vi "简易流程调试界面.vi"() -> ()   [LabVIEW 2016, in "斯坦道氨氮.lvlib"]
uses:
  <userlib>/_OpenG.lib/array/array.llb/Sort 1D Array (I32)__ogtk.vi
  <vilib>/Plasmionique/MB Master/MB_Master/MB_Master.lvclass
panel:
  in  "停止":bool
  out "故障状态":string
  out "告警状态":string
  out "工作状态":string
  in  "单步测试":bool
  out "注射器温度":sgl
  out "消解温度":sgl
  out "ADC":sgl
  out "F3":sgl format="%#.6f"
  out "F2":sgl format="%#.6f"
  out "F1":sgl format="%#.6f"
  out "F0":sgl format="%#.6f"
  in  "启动":bool
  in  "简易流程":u16(ring)
  in  "参数下拉列表":u16(ring)
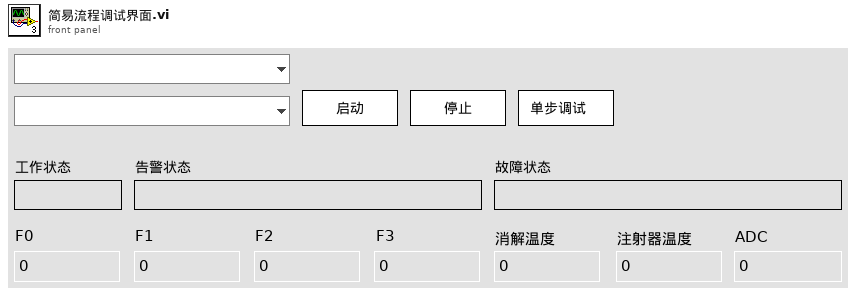
[diagram p1: front panel]
types:
  T1 = typedef "LVStringsAndValuesArrayTypeDef_U16.ctl" = cluster{"String":string, "Value":u16}[]
  T2 = cluster{"系统时间":timestamp, "工作状态":u16, "测量模式":enum16{"待机", "连续模式", "周期模式", "定点模式", "受控模式", "手动模式"}, "告警代码":u16, "故障代码":u16, "日志代码":u16, "软件版本":u16, "F0":sgl, "F1":sgl, "F2":sgl, "F3":sgl, "T":sgl, "H":sgl, "id":u16, "flowid":u16, "量程":u16, "总磷控温温度1":sgl, "营养盐控温温度2":sgl, "ADC":sgl}
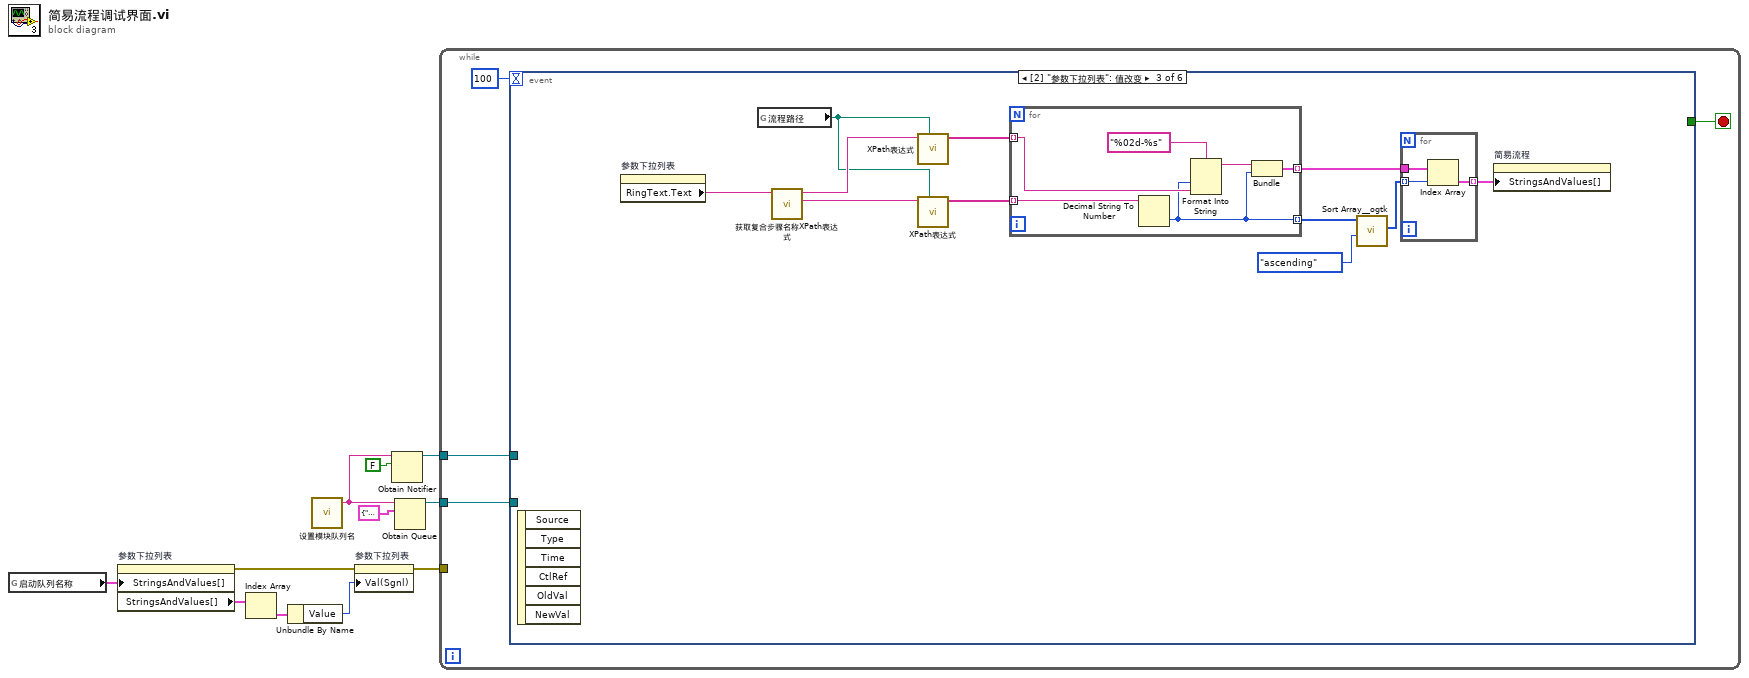
[diagram p0: block diagram]
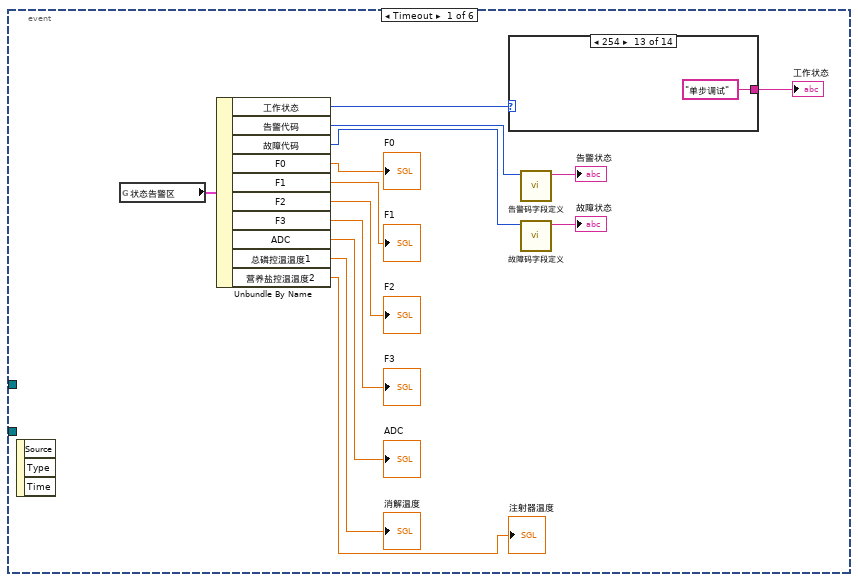
[diagram p2: hidden frame]
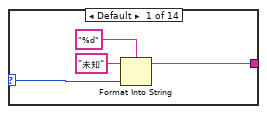
[diagram p3: hidden frame]
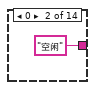
[diagram p4: hidden frame]
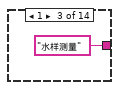
[diagram p5: hidden frame]
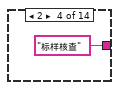
[diagram p6: hidden frame]
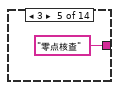
[diagram p7: hidden frame]
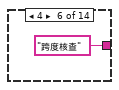
[diagram p8: hidden frame]
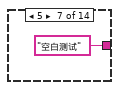
[diagram p9: hidden frame]
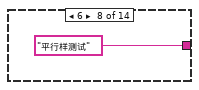
[diagram p10: hidden frame]
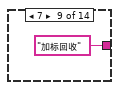
[diagram p11: hidden frame]
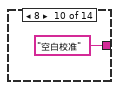
[diagram p12: hidden frame]
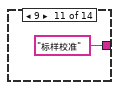
[diagram p13: hidden frame]
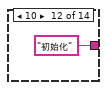
[diagram p14: hidden frame]
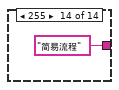
[diagram p15: hidden frame]
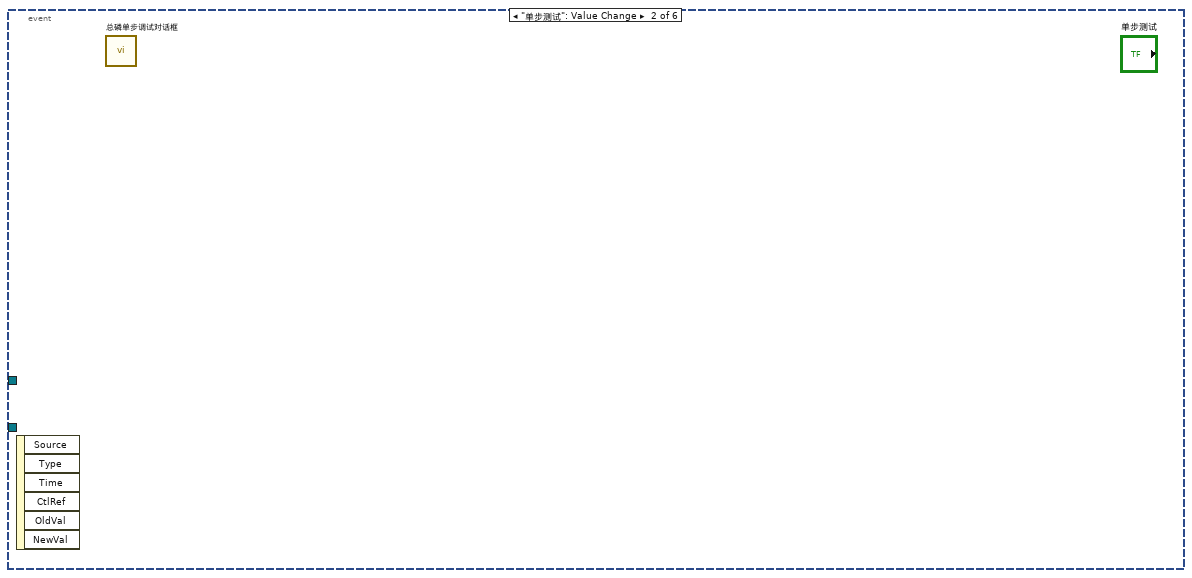
[diagram p16: hidden frame]
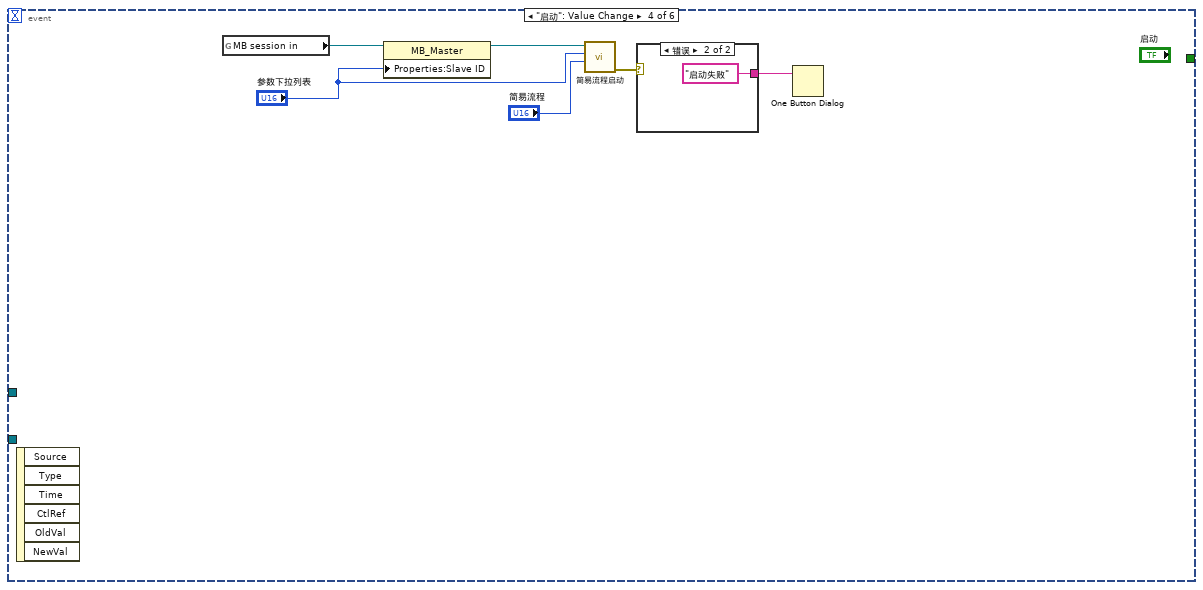
[diagram p17: hidden frame]
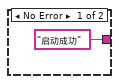
[diagram p18: hidden frame]
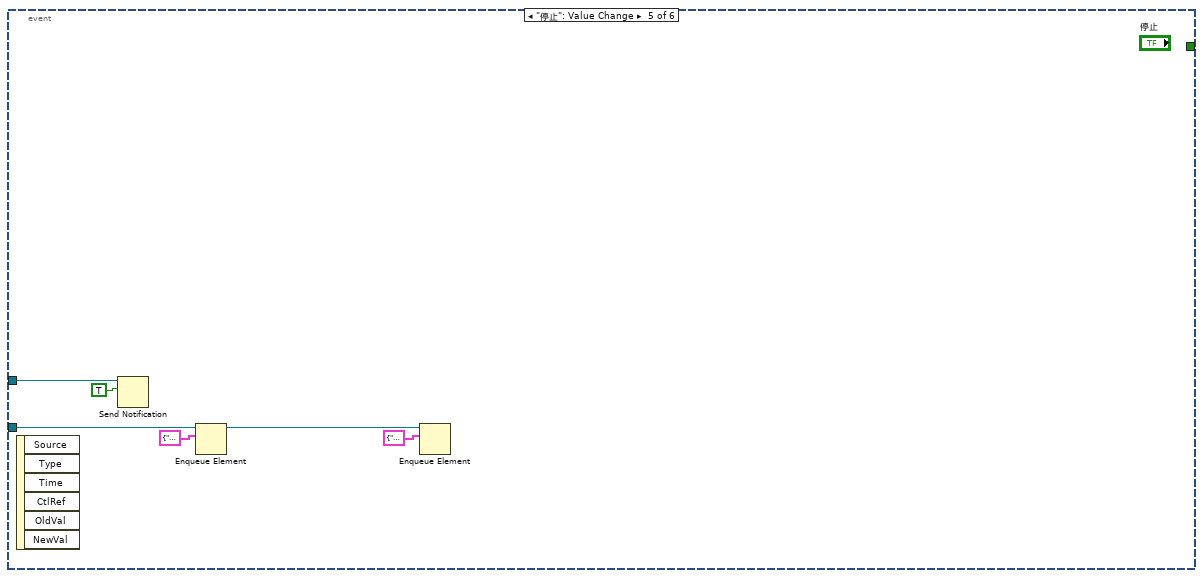
[diagram p19: hidden frame]
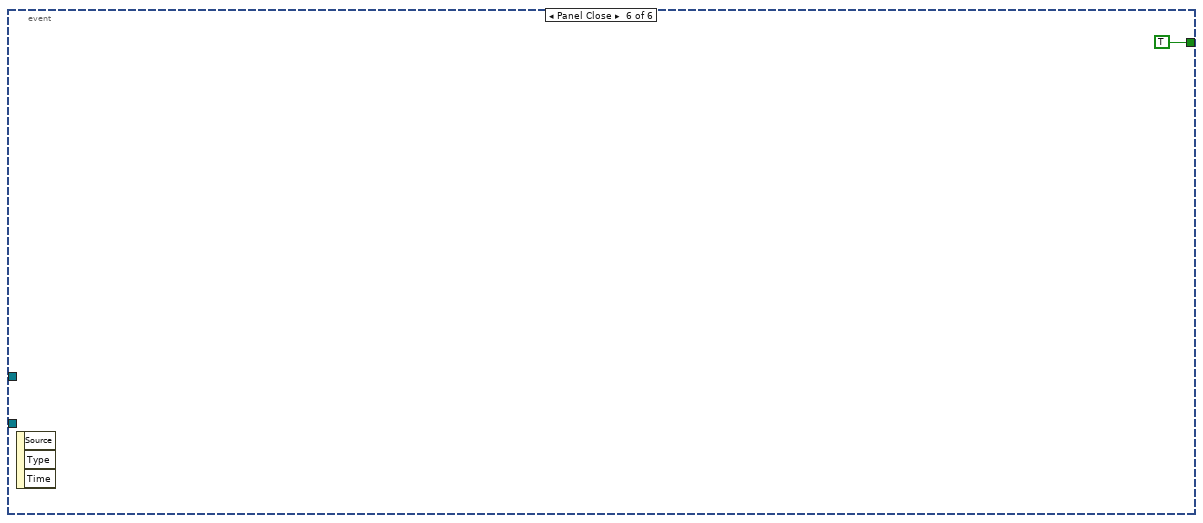
[diagram p20: hidden frame]
diagram:
  n1 = global read "总磷总氮断电保存全局变量.vi" "启动队列名称"() -> (w6:cluster{"String":string, "Value":u16}[])
  n2 = property on="参数下拉列表" class="Ring (严格)"("StringsAndValues[]"=w6) -> (error out=w7:errorcluster, "StringsAndValues[]"=w10:T1)  [unwired: 2 in, 1 out]
  n3 = Index Array(array=w10) -> (element=w9:cluster{"String":string, "Value":u16})  [unwired: 1 in]
  n4 = Unbundle By Name(w9) -> ("Value"=w8:u16)
  n5 = call "设置模块队列名.vi"() -> ("Msg"=w3:string)  [unwired: 5 in]
  n6 = property on="参数下拉列表" class="Ring (严格)"(error in=w7, "Val(Sgnl)"=w8) -> (error out=w11:errorcluster)  [unwired: 1 in, 1 out]
  n7 = Obtain Notifier(name (unnamed)=w3, notification data type=FALSE) -> (notifier out=w2:refnum<notifier>)  [unwired: 2 in, 2 out]
  n8 = Obtain Queue(name (unnamed)=w3, element data type=cluster{"命令":string, "data":variant} {"命令"="", "data"=variant}) -> (queue out=w1:refnum<queue>)  [unwired: 3 in, 2 out]
  n9 = while {
    tunnel: w11 -> [_]
    tunnel: w2 -> [w13]
    tunnel: w1 -> [w12]
    stop <- w15 stop-if-true
    n10 = event shown="[2] \"参数下拉列表\": 值改变" {
      selector: _ -> [_ _ _ _ _ _]
      dyn-events: _ -> [_ _ _ _ _ _]
      timeout: 100 -> [_ _ _ _ _ _]
      tunnel: [_ _ _ _ _ TRUE] -> w15
      tunnel: w13 -> [_ _ _ _ w76 _]
      tunnel: w12 -> [_ _ _ _ w75 _]
      event Timeout {
        n11 = event-data() -> ()  [unwired: 1 in, 3 out]
        n12 = global read "VAR总磷总氮全局变量.vi" "状态告警区"() -> (w29:T2)
        n13 = Unbundle By Name(w29) -> ("工作状态"=w21:u16, "告警代码"=w20:u16, "故障代码"=w19:u16, "F0"=→"F0":sgl, "F1"=→"F1":sgl, "F2"=→"F2":sgl, "F3"=→"F3":sgl, "ADC"=→"ADC":sgl, "总磷控温温度1"=→"消解温度":sgl, "营养盐控温温度2"=→"注射器温度":sgl)
        n14 = case shown="254" w21 {
          selector: w21 -> [w30 _ _ _ _ _ _ _ _ _ _ _ _ _]
          tunnel: [w31 "空闲" ("工作状态") "水样测量" ("工作状态") "标样核查" ("工作状态") "零点核查" ("工作状态") "跨度核查" ("工作状态") "空白测试" ("工作状态") "平行样测试" ("工作状态") "加标回收" ("工作状态") "空白校准" ("工作状态") "标样校准" ("工作状态") "初始化" ("工作状态") "单步调试" ("工作状态") "简易流程" ("工作状态")] -> w18
          frame Default {
            n15 = Format Into String(format string="%d" ("格式字符串"), initial string="未知" ("工作状态"), w30) -> (resulting string=w31:string)  [unwired: 1 in, 1 out]
          }
          frame 0 {
          }
          frame 1 {
          }
          frame 2 {
          }
          frame 3 {
          }
          frame 4 {
          }
          frame 5 {
          }
          frame 6 {
          }
          frame 7 {
          }
          frame 8 {
          }
          frame 9 {
          }
          frame 10 {
          }
          frame 254 {
          }
          frame 255 {
          }
        }
        "工作状态" <- w18
        n16 = call "告警码字段定义.vi"("告警代码"=w20) -> ("字符串"=→"告警状态":string)  [unwired: 8 in, 2 out]
        n17 = call "故障码字段定义.vi"("故障代码"=w19) -> ("字符串"=→"故障状态":string)  [unwired: 10 in]
      }
      event "单步测试": Value Change {
        n18 = event-data() -> ()  [unwired: 1 in, 6 out]
        n19 = call "总磷单步调试对话框.vi"() -> ()  [unwired: 12 in]
      }
      event "参数下拉列表": Value Change {
        n20 = event-data() -> ()  [unwired: 1 in, 6 out]
        n21 = property on="参数下拉列表" class="Ring (严格)"() -> ("RingText.Text"=w57:string)  [unwired: 2 in, 2 out]
        n22 = global read "总磷总氮断电保存全局变量.vi" "流程路径"() -> (w52:path)
        n23 = call "获取复合步骤名称XPath表达式.vi"("查询参数"=w57) -> ("FlowId"=w55:string, "name"=w56:string)  [unwired: 9 in]
        n24 = call "XPath表达式.vi"("添加的路径"=w52, "XPath expression"=w56) -> ("数组"=w54:string[])  [unwired: 9 in]
        n25 = call "XPath表达式.vi"("添加的路径"=w52, "XPath expression"=w55) -> ("数组"=w53:string[])  [unwired: 9 in]
        n26 = for {
          tunnel: w54 -> [w63] mode=indexing
          tunnel: w53 -> [w66] mode=indexing
          tunnel: [w65] -> w49 mode=indexing
          tunnel: [w61] -> w51 mode=indexing
          n27 = Decimal String To Number(string=w66) -> (number=w61:i32)  [unwired: 2 in, 1 out]
          n28 = Format Into String(format string="%02d-%s" ("格式字符串"), w61, w63) -> (resulting string=w62:string)  [unwired: 2 in, 1 out]
          n29 = Bundle(w62, w61) -> (w65:cluster{string, i32})  [unwired: 1 in]
        }
        n30 = call-poly <userlib>:"Sort Array__ogtk.vi"("Order"=enum16{"ascending", "descending"}."ascending", "Array in"=w51) -> ("Sorted Pointers"=w48:i32[])  [unwired: 8 in, 1 out]
        n31 = for {
          tunnel: w49 -> [w60]
          tunnel: w48 -> [w59] mode=indexing
          tunnel: [w58] -> w47 mode=indexing
          n32 = Index Array(array=w60, index=w59) -> (element=w58:cluster{string, i32})
        }
        n33 = property on="简易流程" class="Ring (严格)"("StringsAndValues[]"=w47) -> ()  [unwired: 2 in, 2 out]
      }
      event "启动": Value Change {
        n34 = event-data() -> ()  [unwired: 1 in, 6 out]
        n35 = global read "VAR总磷总氮全局变量.vi" "MB session in"() -> (w70:refnum<class "MB_Master.lvclass">)
        n36 = property class="MB_Master"(reference=w70, "Properties:Slave ID"="参数下拉列表") -> (reference out=w69:refnum<class "MB_Master.lvclass">)  [unwired: 1 in, 1 out]
        n37 = call "简易流程启动.vi"("简易流程"="简易流程", "参数Id"="参数下拉列表", "MB session in"=w69) -> ("error out"=w72:errorcluster)  [unwired: 7 in, 1 out]
        n38 = case shown="错误" w72 {
          tunnel: ["启动成功" "启动失败"] -> w71
          frame No Error {
          }
          frame Error {
          }
        }
        n39 = One Button Dialog(message=w71) -> ()  [unwired: 1 in, 1 out]
      }
      event "停止": Value Change {
        n40 = event-data() -> ()  [unwired: 1 in, 6 out]
        n41 = Send Notification(notification=TRUE ("通知"), notifier=w76) -> ()  [unwired: 1 in, 2 out]
        n42 = Enqueue Element(queue=w75, element=cluster{"命令":string, "data":variant} {"命令"="启动", "data"=variant(cluster{"站号":u16, "控制命令输出":u16[]} {"站号"=1, "控制命令输出"=[2816]})} ("元素")) -> (queue out=w78:refnum<queue>)  [unwired: 2 in, 2 out]
        n43 = Enqueue Element(queue=w78, element=cluster{"命令":string, "data":variant} {"命令"="启动", "data"=variant(cluster{"站号":u16, "控制命令输出":u16[]} {"站号"=2, "控制命令输出"=[2816]})} ("元素")) -> ()  [unwired: 2 in, 3 out]
      }
      event Panel Close {
        n44 = event-data() -> ()  [unwired: 1 in, 3 out]
      }
    }
  }
